vi "Set Current Caster Angle_Frame.vi"(7 "ignore (F)":bool, 8 "error in (no error)":errorcluster, 10 "current caster angle (rad)":dbl, 11 "wheel in":refnum<class "NI_Robotics_Wheel.lvclass">) -> (0 "error out":errorcluster, 3 "wheel out":refnum<class "NI_Robotics_Wheel.lvclass">)   [LabVIEW 2017, in "NI_Robotics_Wheel.lvclass"]
uses:
  <vilib>/robotics/Steering/Wheel/NI_Robotics_Wheel.lvclass
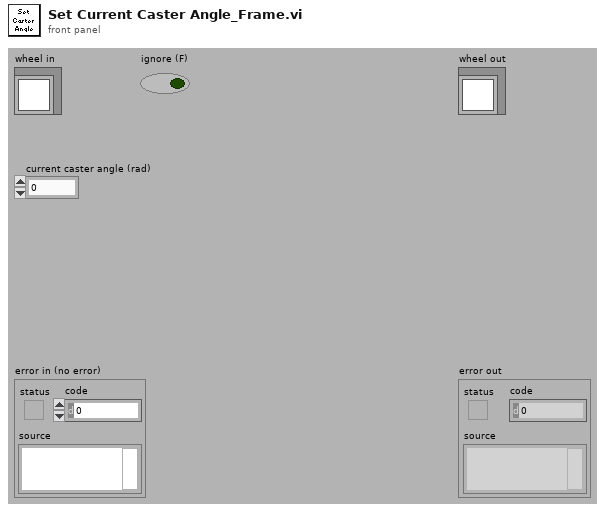
[diagram p1: front panel]
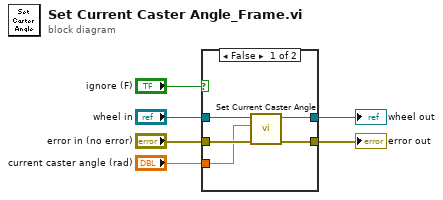
[diagram p0: block diagram]
diagram:
  n1 = case shown="False" "ignore (F)" {
    tunnel: "wheel in" -> [w11 w13]
    tunnel: [w10 w13] -> w5
    tunnel: "error in (no error)" -> [w9 w12]
    tunnel: [w8 w12] -> w3
    tunnel: "current caster angle (rad)" -> [w7 _]
    frame False {
      n2 = call-dynamic "Set Current Caster Angle.vi"("error in (no error)"=w9, "current caster angle (rad)"=w7, "wheel in"=w11) -> ("error out"=w8:errorcluster, "wheel out"=w10:refnum<class "NI_Robotics_Wheel.lvclass">)  [unwired: 7 in]
    }
    frame True {
    }
  }
  "error out" <- w3
  "wheel out" <- w5
